vi "GetAutoData.vi"   [LabVIEW 2017]
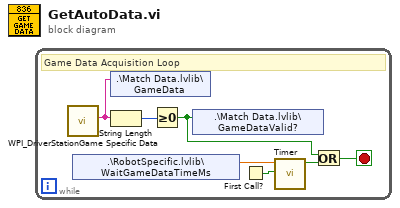
[diagram p0: block diagram]
diagram:
  n1 = while {
    stop <- w4 stop-if-true
    # "Game Data Acquisition Loop"
    n2 = call <vilib>:"WPI_DriverStationGame Specific Data.vi"() -> ("Game Specific Data"=w2:string)  [unwired: 11 in]
    n3 = shared-variable ".\\RobotSpecific.lvlib\\WaitGameDataTimeMs"() -> (w6:dbl)  [unwired: 1 in, 1 out]
    n4 = shared-variable ".\\Match Data.lvlib\\GameData"(w2) -> ()  [unwired: 1 in, 1 out]
    n5 = String Length(string=w2) -> (length=w7:i32)
    n6 = Greater Or Equal To 0?(x=w7) -> (x >= 0?=w1:bool)
    n7 = shared-variable ".\\Match Data.lvlib\\GameDataValid?"(w1) -> ()  [unwired: 1 in, 1 out]
    n8 = First Call?() -> (First Call?: T/F=w5:bool)
    n9 = call <userlib>:"Timer.vi"("Start"=w5, "Time (ms)"=w6) -> ("Time Expired?"=w3:bool)  [unwired: 7 in, 2 out]
    n10 = Or(x=w1, y=w3) -> (x .or. y?=w4:bool)
  }
